vi "FGV_PowerAmplifier_Transmit.vi"(7 "Write?":bool, 8 "error in":errorcluster caption="错误输入", 11 "Transmit":string[][](array[string])) -> (0 "error out":errorcluster caption="错误输出", 3 "Transmit out":string[][](array[string]))   [LabVIEW 2020]
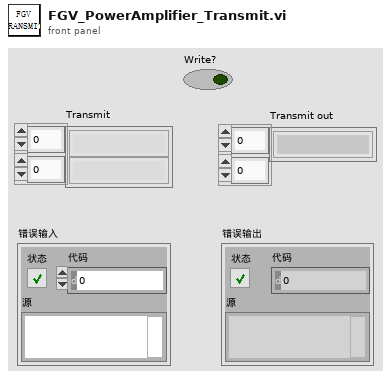
[diagram p1: front panel]
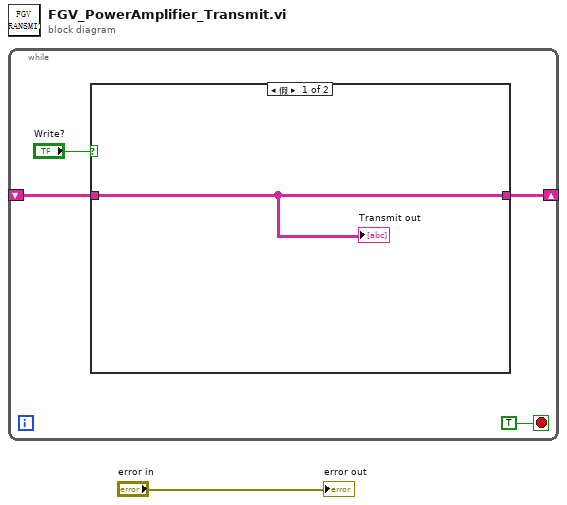
[diagram p0: block diagram]
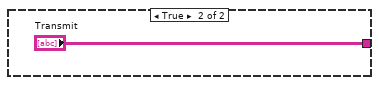
[diagram p2: hidden frame]
diagram:
  n1 = while {
    shift-right: [w4] -> _
    shift-left: _ -> [w3]
    stop <- TRUE stop-if-true
    n2 = case shown="假" "Write?" {
      tunnel: [w6 "Transmit"] -> w4
      tunnel: w3 -> [w6 _]
      frame False {
        "Transmit out" <- w6
      }
      frame True {
      }
    }
  }
  "error out" <- "error in"
